vi "SetChannelXConfig.vi"(1 "Error In":errorcluster, 2 "Channel1":T1={"AutoLevel"=FALSE, "Thresold"=1.0, "Active Edge"=1, "Impedance "=1000000.0, "Voltage Range"=5.0} {"Impedance" items=["50"=50.0, "1E+6"=1000000.0]; "Active Edge" items=["Positive", "Negative"]}, 3 "Channel (1: Channel 1)":i32(ring)=1 items=["Channel 1"=1, "Channel 2"=2], 4 "VISA Ressource":string) -> (0 "Error Out":errorcluster)   [LabVIEW 2014]
uses:
  Channel.ctl
  <instrlib>/Agilent 532XX Series/Public/Configure/Configure Channel (Auto Threshold Voltage).vi
  <instrlib>/Agilent 532XX Series/Public/Configure/Configure Channel (Basic).vi
  <instrlib>/Agilent 532XX Series/Public/Configure/Configure Channel (Slop).vi
  <instrlib>/Agilent 532XX Series/Public/Configure/Configure Channel (Threshold Voltage).vi
  <instrlib>/Agilent 532XX Series/Public/Configure/Configure Channel (Voltage Range).vi
  <instrlib>/Agilent 532XX Series/Agilent 532XX Series.lvlib
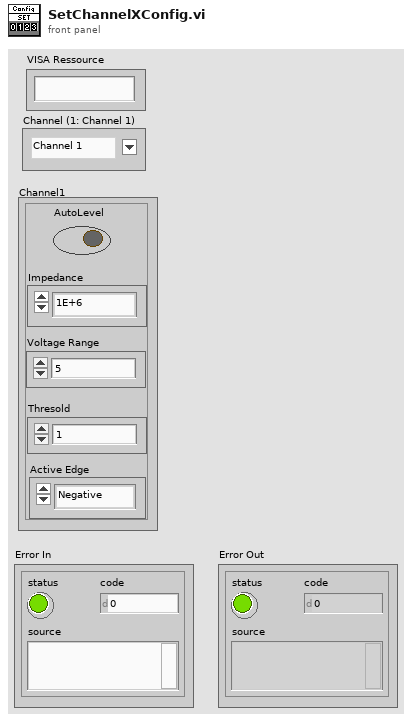
[diagram p1: front panel]
types:
  T1 = typedef "Channel.ctl" = cluster{"AutoLevel":bool, "Thresold":dbl, "Active Edge":i32, "Impedance ":dbl, "Voltage Range":dbl}
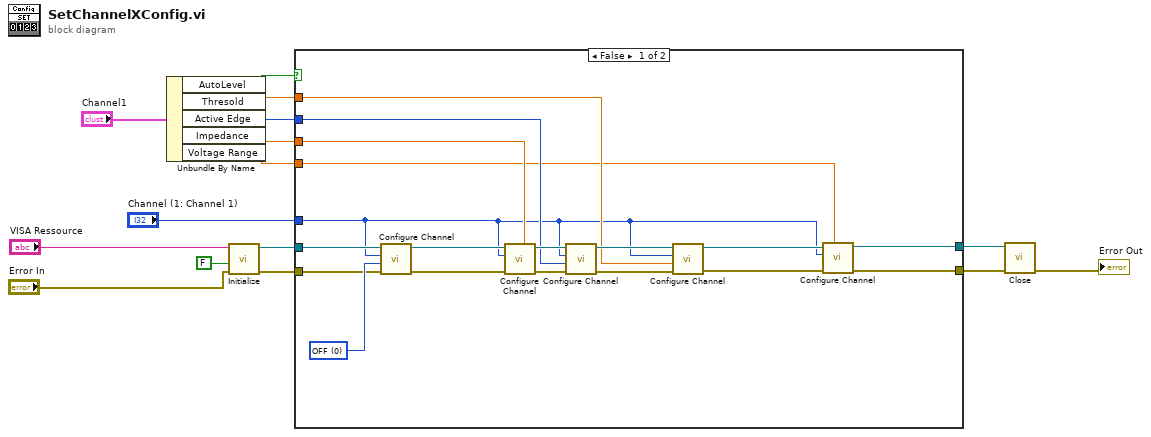
[diagram p0: block diagram]
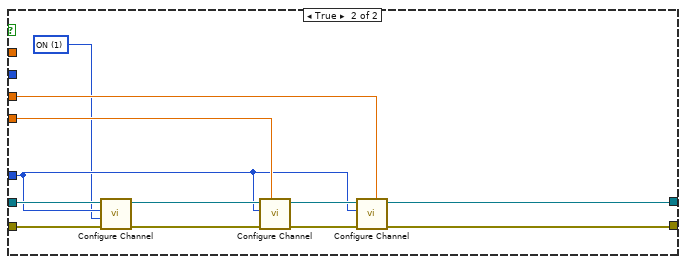
[diagram p2: hidden frame]
diagram:
  n1 = Unbundle By Name("Channel1") -> ("AutoLevel"=w9:bool, "Thresold"=w3:dbl, "Active Edge"=w4:i32, "Impedance"=w8:dbl, "Voltage Range"=w7:dbl)
  n2 = call <instrlib>:"Initialize.vi"("error in (no error)"="Error In", "Reset (True)"=FALSE, "VISA resource name"="VISA Ressource") -> ("error out"=w11:errorcluster, "VISA resource name out"=w12:refnum<visa-resource-name>)  [unwired: 7 in]
  n3 = case shown="False" w9 {
    tunnel: "Channel (1: Channel 1)" -> [w18 w37]
    tunnel: w12 -> [w32 w45]
    tunnel: w11 -> [w31 w44]
    tunnel: w8 -> [w28 w43]
    tunnel: w7 -> [w19 w38]
    tunnel: [w17 w36] -> w6
    tunnel: [w16 w35] -> w5
    tunnel: w4 -> [w25 _]
    tunnel: w3 -> [w22 _]
    frame False {
      w33 = 0 items=["OFF", "ON", "ONCE"] ("Enable Auto-leveling (1: ON)")
      n4 = call-poly <instrlib>:"Configure Channel.vi"("error in (no error)"=w31, "Enable Auto-leveling (1: ON)"=w33, "Channel (1: Channel 1)"=w18, "VISA resource name"=w32) -> ("error out"=w30:errorcluster, "VISA resource name out"=w29:refnum<visa-resource-name>)  [unwired: 6 in]
      n5 = call-poly <instrlib>:"Configure Channel.vi"("Impedance (1E+6 Ohm)"=w28, "error in (no error)"=w30, "Channel (1: Channel 1)"=w18, "VISA resource name"=w29) -> ("error out"=w27:errorcluster, "VISA resource name out"=w26:refnum<visa-resource-name>)  [unwired: 6 in]
      n6 = call-poly <instrlib>:"Configure Channel.vi"("error in (no error)"=w27, "Active Edge (1: Negative)"=w25, "Channel (1: Channel 1)"=w18, "VISA resource name"=w26) -> ("error out"=w24:errorcluster, "VISA resource name out"=w23:refnum<visa-resource-name>)  [unwired: 6 in]
      n7 = call-poly <instrlib>:"Configure Channel.vi"("error in (no error)"=w24, "Threshold Voltage (0 V)"=w22, "Channel (1: Channel 1)"=w18, "VISA resource name"=w23) -> ("error out"=w20:errorcluster, "VISA resource name out"=w21:refnum<visa-resource-name>)  [unwired: 6 in]
      n8 = call-poly <instrlib>:"Configure Channel.vi"("Voltage Range (5V)"=w19, "error in (no error)"=w20, "Channel (1: Channel 1)"=w18, "VISA resource name"=w21) -> ("error out"=w16:errorcluster, "VISA resource name out"=w17:refnum<visa-resource-name>)  [unwired: 6 in]
    }
    frame True {
      w34 = 1 items=["OFF", "ON", "ONCE"] ("Enable Auto-leveling (1: ON)")
      n9 = call-poly <instrlib>:"Configure Channel.vi"("error in (no error)"=w44, "Enable Auto-leveling (1: ON)"=w34, "Channel (1: Channel 1)"=w37, "VISA resource name"=w45) -> ("error out"=w41:errorcluster, "VISA resource name out"=w42:refnum<visa-resource-name>)  [unwired: 6 in]
      n10 = call-poly <instrlib>:"Configure Channel.vi"("Voltage Range (5V)"=w38, "error in (no error)"=w41, "Channel (1: Channel 1)"=w37, "VISA resource name"=w42) -> ("error out"=w39:errorcluster, "VISA resource name out"=w40:refnum<visa-resource-name>)  [unwired: 6 in]
      n11 = call-poly <instrlib>:"Configure Channel.vi"("Impedance (1E+6 Ohm)"=w43, "error in (no error)"=w39, "Channel (1: Channel 1)"=w37, "VISA resource name"=w40) -> ("error out"=w35:errorcluster, "VISA resource name out"=w36:refnum<visa-resource-name>)  [unwired: 6 in]
    }
  }
  n12 = call <instrlib>:"Close.vi"("error in (no error)"=w5, "VISA resource name"=w6) -> ("error out"=→"Error Out":errorcluster)  [unwired: 9 in]
